vi "Initialise piezo.vi"() -> (0 "Piezo error out":errorcluster, 3 "Piezo handle":i32)   [LabVIEW 2017]
uses:
  <instrlib>/Thorlabs_MDT69xB/Thorlabs_MDT69xB.lvlib
panel:
  in  "VISA resource name":refnum<visa-resource-name>="COM5"
  # "Piezo is on COM5"
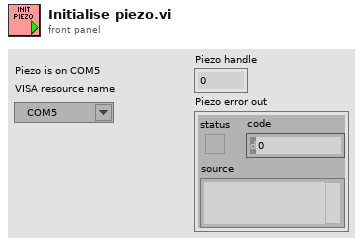
[diagram p1: front panel]
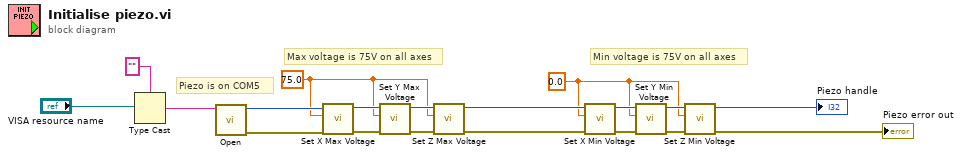
[diagram p0: block diagram]
diagram:
  w10 = 75.0 ("x max Voltage")
  w3 = 0.0 ("x min Voltage")
  # "Min voltage is 75V on all axes"
  # "Max voltage is 75V on all axes"
  # "Piezo is on COM5"
  n1 = Type Cast(type="", x="VISA resource name") -> (*(type *) &x=w17:string)
  n2 = call <instrlib>:"Open.vi"("Serial Port"=w17) -> ("error out"=w16:errorcluster, "hDevice"=w15:i32)  [unwired: 8 in, 1 out]
  n3 = call <instrlib>:"Set X Max Voltage.vi"("error in (no error)"=w16, "x max Voltage"=w10, "hdl in"=w15) -> ("error out"=w14:errorcluster, "hdl"=w13:i32)  [unwired: 7 in]
  n4 = call <instrlib>:"Set Y Max Voltage.vi"("error in (no error)"=w14, "y max Voltage"=w10, "hdl in"=w13) -> ("error out"=w12:errorcluster, "hdl"=w11:i32)  [unwired: 7 in]
  n5 = call <instrlib>:"Set Z Max Voltage.vi"("error in (no error)"=w12, "z max Voltage"=w10, "hdl in"=w11) -> ("error out"=w8:errorcluster, "hdl"=w9:i32)  [unwired: 7 in]
  n6 = call <instrlib>:"Set X Min Voltage.vi"("error in (no error)"=w8, "x min Voltage"=w3, "hdl in"=w9) -> ("error out"=w7:errorcluster, "hdl"=w6:i32)  [unwired: 7 in]
  n7 = call <instrlib>:"Set Y Min Voltage.vi"("error in (no error)"=w7, "y min Voltage"=w3, "hdl in"=w6) -> ("error out"=w4:errorcluster, "hdl"=w5:i32)  [unwired: 7 in]
  n8 = call <instrlib>:"Set Z Min Voltage.vi"("error in (no error)"=w4, "z min Voltage"=w3, "hdl in"=w5) -> ("error out"=→"Piezo error out":errorcluster, "hdl"=→"Piezo handle":i32)  [unwired: 7 in]
